vi "FILE PATH CREATION.vi"(8 "error in (no error)":errorcluster, 11 "Fill Name":string) -> (0 "error out":errorcluster, 3 "dup directory path":path)   [LabVIEW 2023]
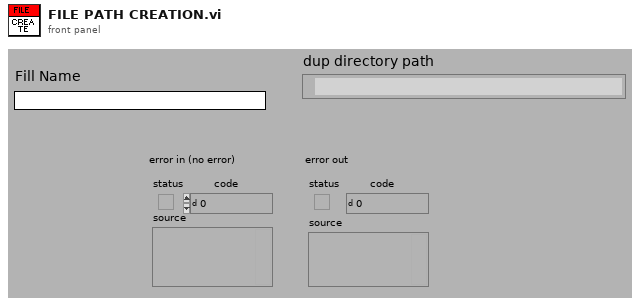
[diagram p1: front panel]
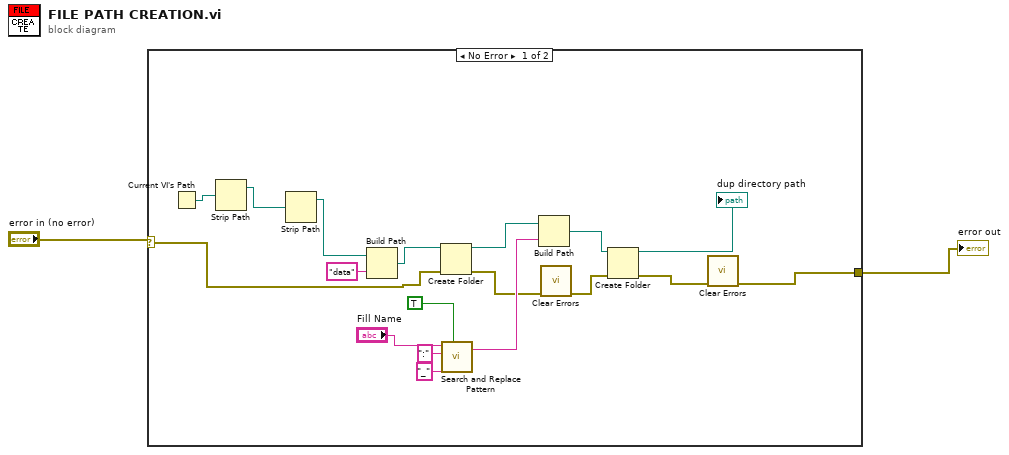
[diagram p0: block diagram]
diagram:
  n1 = case shown="No Error" "error in (no error)" {
    selector: "error in (no error)" -> [w7 _]
    tunnel: [w5 _] -> w1
    frame No Error {
      n2 = Current VI's Path() -> (path=w19:path)
      n3 = Strip Path(path=w19) -> (stripped path=w4:path)  [unwired: 1 out]
      n4 = Strip Path(path=w4) -> (stripped path=w3:path)  [unwired: 1 out]
      n5 = Build Path(base path=w3, name or relative path="data") -> (appended path=w18:path)
      n6 = Create Folder(path (use dialog)=w18, error in=w7) -> (created path=w13:path, error out=w10:errorcluster)  [unwired: 1 in, 1 out]
      n7 = call <vilib>:"Search and Replace Pattern.vi"("string"="Fill Name", "regular expression (\"\")"=":" ("regular expression (\"\")"), "replace string (\"\")"="_" ("replace string (\"\")"), "replace all? (F)"=TRUE) -> ("result string"=w12:string)  [unwired: 1 in, 1 out]
      n8 = Build Path(base path=w13, name or relative path=w12) -> (appended path=w11:path)
      n9 = call <vilib>:"Clear Errors.vi"("error in (no error)"=w10) -> ("error out"=w9:errorcluster)  [unwired: 5 in, 1 out]
      n10 = Create Folder(path (use dialog)=w11, error in=w9) -> (created path=→"dup directory path":path, error out=w6:errorcluster)  [unwired: 1 in, 1 out]
      n11 = call <vilib>:"Clear Errors.vi"("error in (no error)"=w6) -> ("error out"=w5:errorcluster)  [unwired: 5 in, 1 out]
    }
    frame Error {
    }
  }
  "error out" <- w1
